vi "Extract Project Strings.vi"(8 "error in (no error)":errorcluster, 11 "New Project Wizard in":refnum<class "Update Project Wizard.lvclass">) -> (0 "error out":errorcluster, 3 "New Project Wizard out":refnum<class "Update Project Wizard.lvclass">)   [LabVIEW 2013, in "SET Project Editor.lvlib" / "Update Project Wizard.lvclass"]
uses:
  Update Project Wizard.lvclass
  Update Project Wizard.lvclass/Update Project Wizard.ctl
  SET Project Data/Project Data Class/Project Data.lvclass
  SET Project Data/Resource Data Class/Resource Data.lvclass
  Lib/Printf/Messages/General/LV_Printf Msg.lvclass
  SET Project Data/VI Class/VI Data.lvclass
  SET Project Data/Menu Class/Menu Data.lvclass
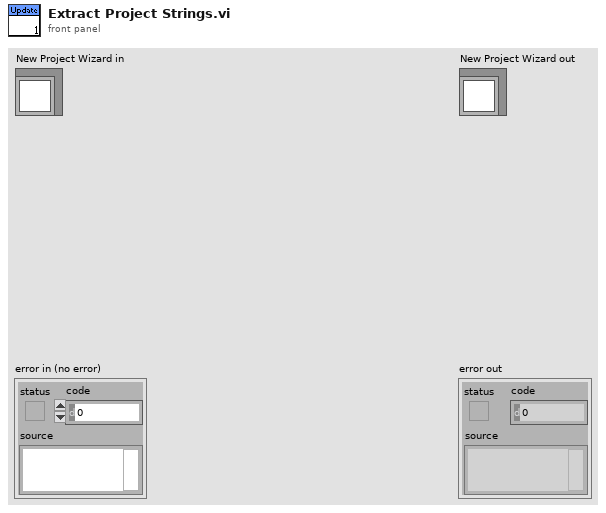
[diagram p1: front panel]
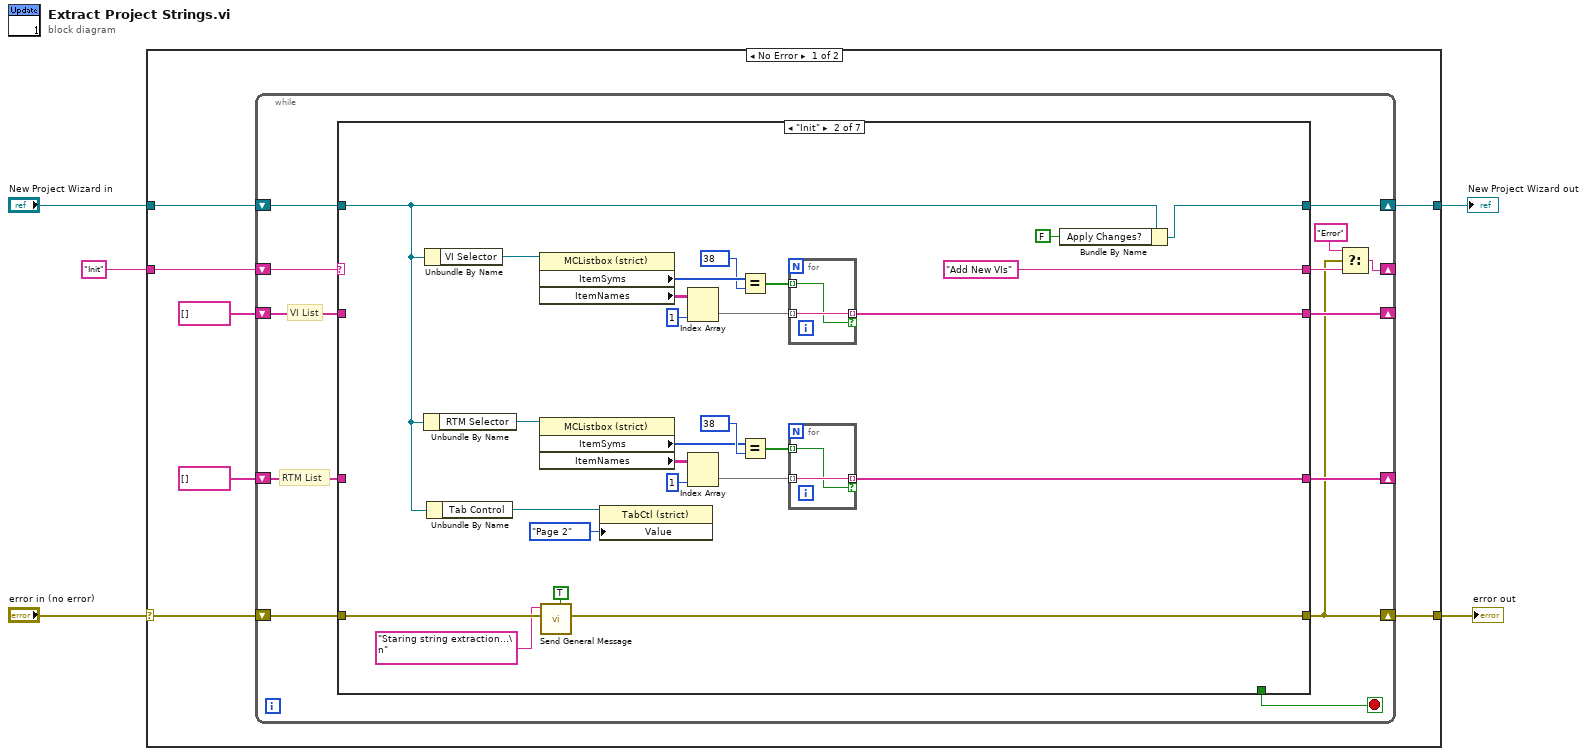
[diagram p0: block diagram]
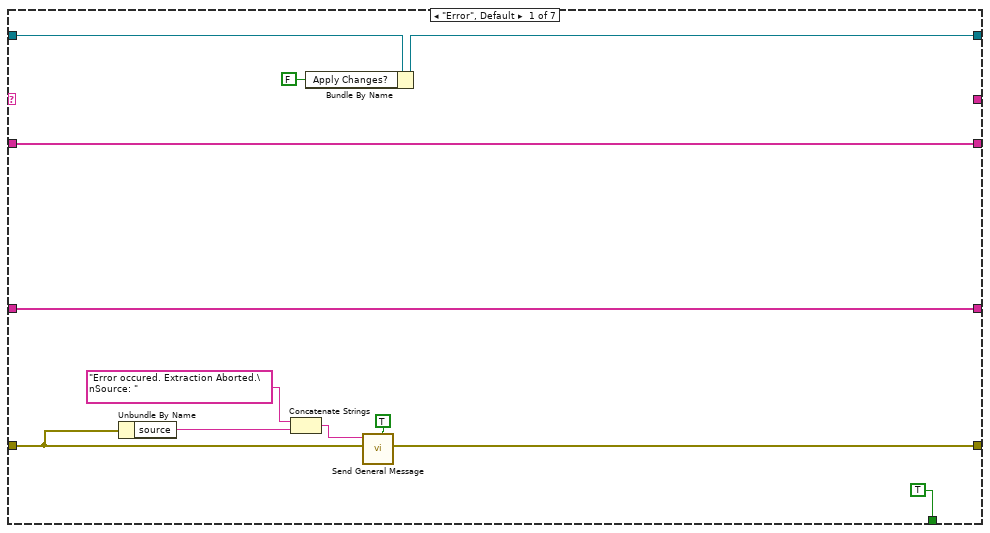
[diagram p2: hidden frame]
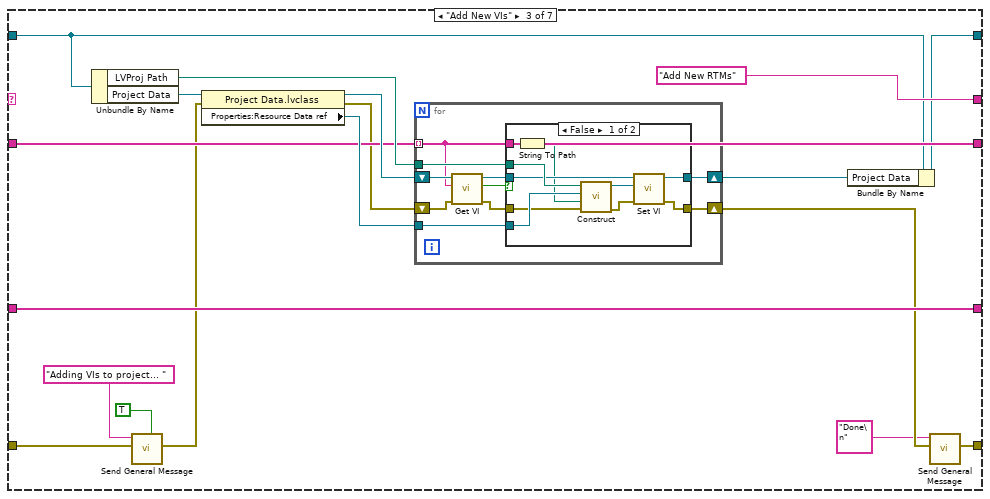
[diagram p3: hidden frame]
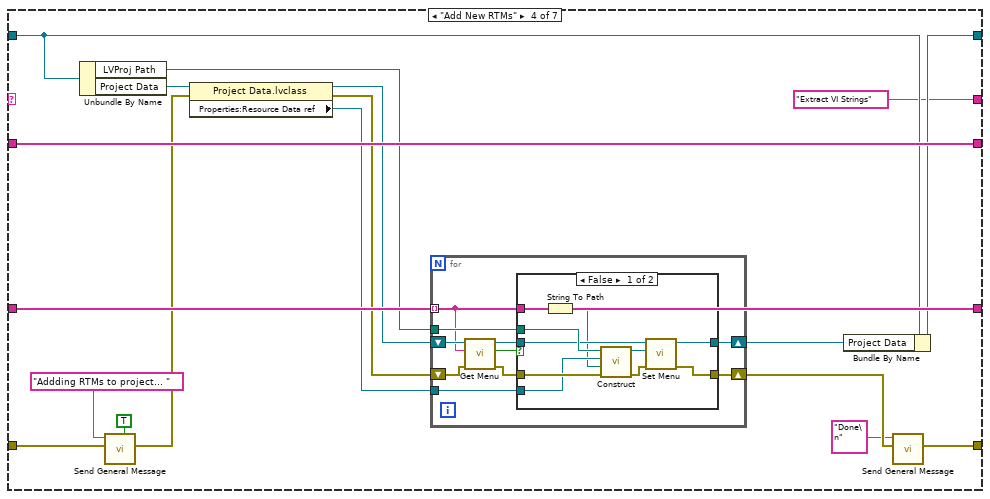
[diagram p5: hidden frame]
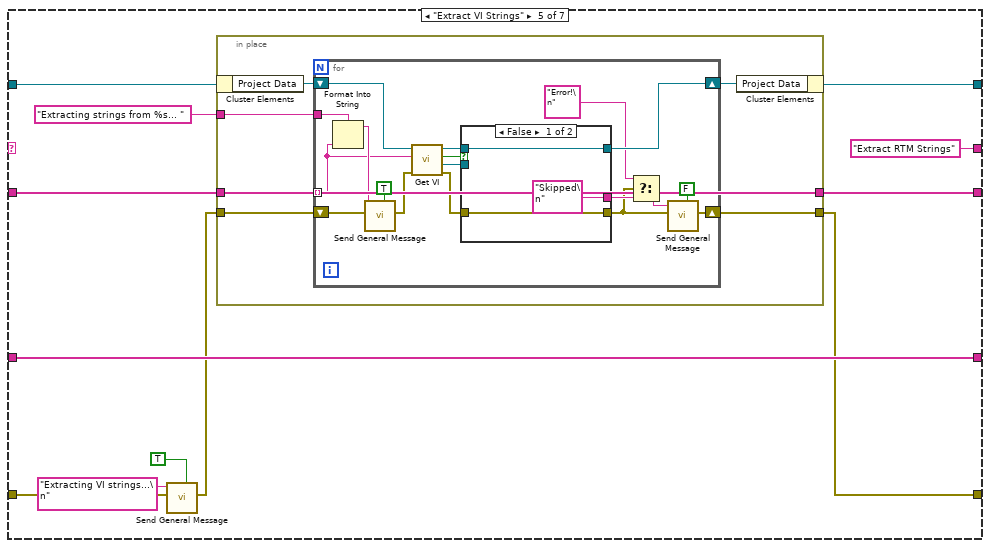
[diagram p7: hidden frame]
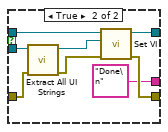
[diagram p8: hidden frame]
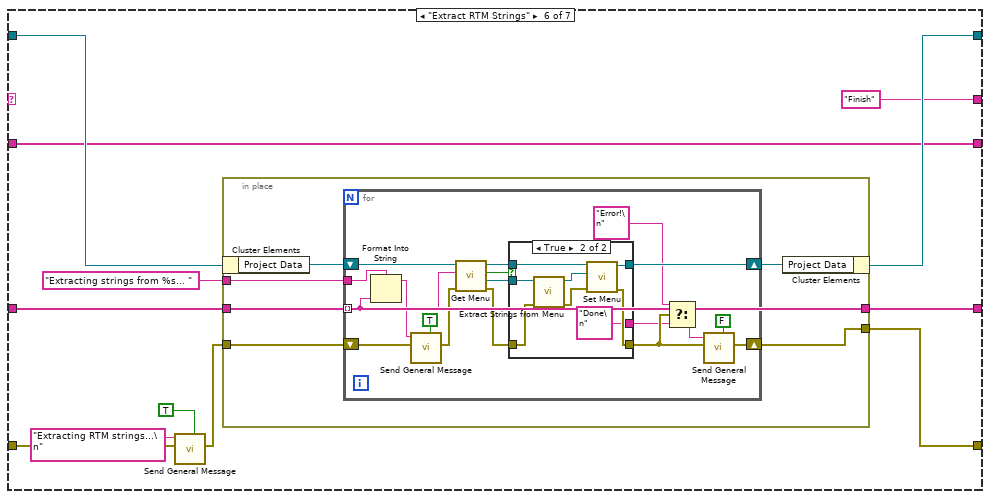
[diagram p9: hidden frame]
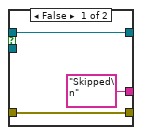
[diagram p10: hidden frame]
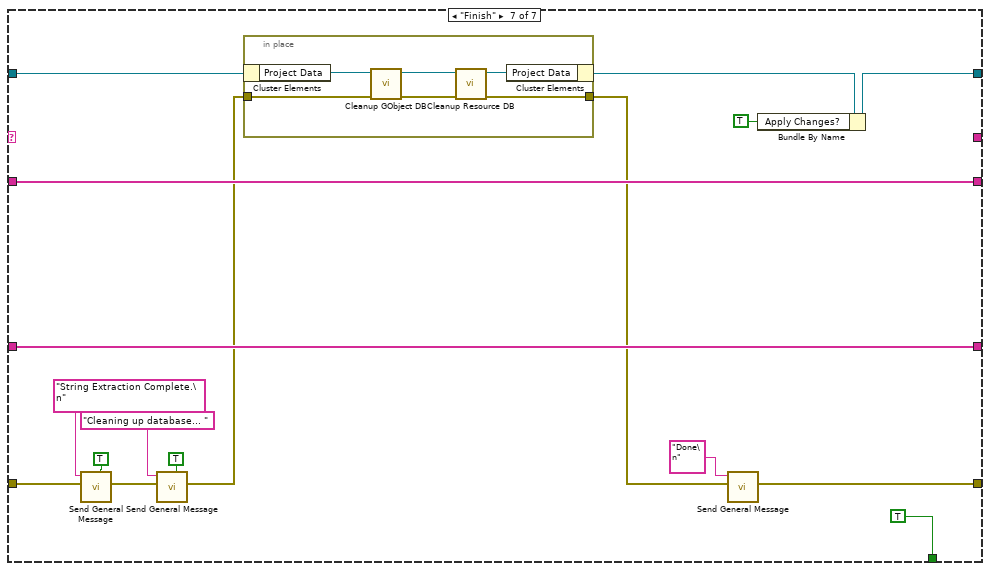
[diagram p11: hidden frame]
diagram:
  n1 = case shown="No Error" "error in (no error)" {
    selector: "error in (no error)" -> [w7 w266]
    tunnel: [w6 w266] -> w1
    tunnel: [w8 w265] -> w2
    tunnel: "New Project Wizard in" -> [w12 w265]
    tunnel: "Init" -> [w11 _]
    frame No Error {
      n2 = while {
        shift-right: [w14] -> _
        shift-left: w11 -> [w25]
        shift-right: [w19] -> w8
        shift-left: w12 -> [w24]
        shift-right: [w23] -> _
        shift-left: string[] [] -> [w22]
        shift-right: [w21] -> _
        shift-left: string[] [] -> [w20]
        shift-right: [w15] -> w6
        shift-left: w7 -> [w17]
        stop <- w18 stop-if-true
        # "RTM List"
        # "VI List"
        n3 = case shown="\"Init\"" w25 {
          tunnel: w24 -> [w28 w38 w78 w118 w159 w206 w255]
          tunnel: [w37 w56 w80 w123 w157 w201 w258] -> w23
          tunnel: w22 -> [w37 _ w80 w123 w158 w201 w258]
          tunnel: [w36 w48 w81 w124 w154 w202 w257] -> w21
          tunnel: w20 -> [w36 _ w81 w124 w154 w203 w257]
          tunnel: [w27 w39 w77 w117 w156 w205 w243] -> w19
          tunnel: [_ "Add New VIs" "Add New RTMs" "Extract VI Strings" "Extract RTM Strings" "Finish" _] -> w16
          tunnel: [TRUE _ _ _ _ _ TRUE] -> w18
          tunnel: w17 -> [w32 w44 w74 w114 w152 w197 w254]
          tunnel: [w33 w41 w70 w110 w153 w200 w246] -> w15
          frame "Error", Default {
            n4 = Unbundle By Name(w32) -> ("source"=w30:string)
            n5 = Concatenate Strings("Error occured. Extraction Aborted.\nSource: ", w30) -> (w29:string)
            n6 = Bundle By Name(cluster=w28, "Apply Changes?"=FALSE) -> (w27:refnum<class "Update Project Wizard.lvclass">)
            n7 = call "Send General Message.vi"("Timestamp in message? (F)"=TRUE, "error in (no error)"=w32, "Message"=w29) -> ("error out"=w33:errorcluster)  [unwired: 8 in]
          }
          frame "Init" {
            n8 = Unbundle By Name(w38) -> ("RTM Selector"=w49:refnum<vi>)
            n9 = Unbundle By Name(w38) -> ("VI Selector"=w59:refnum<vi>)
            n10 = Unbundle By Name(w38) -> ("Tab Control"=w46:refnum<vi>)
            n11 = property class="MCListbox (strict)"(reference=w59) -> ("ItemSyms"=w61:i32[], "ItemNames"=w62:string[][])  [unwired: 1 in, 2 out]
            n12 = property class="MCListbox (strict)"(reference=w49) -> ("ItemSyms"=w52:i32[], "ItemNames"=w51:string[][])  [unwired: 1 in, 2 out]
            n13 = call "Send General Message.vi"("Timestamp in message? (F)"=TRUE, "error in (no error)"=w44, "Message"="Staring string extraction...\n" ("Status")) -> ("error out"=w41:errorcluster)  [unwired: 8 in]
            n14 = property class="TabCtl (strict)"(reference=w46, "Value"=enum32{"Page 1", "Page 2"}."Page 2") -> ()  [unwired: 1 in, 2 out]
            n15 = Index Array(array=w62, index (col)=1 ("disabled index (col)")) -> (element=w58:string[])  [unwired: 1 in]
            n16 = Index Array(array=w51, index (col)=1 ("disabled index (col)")) -> (element=w54:string[])  [unwired: 1 in]
            n17 = Equal?(x=w61, y=38) -> (x = y?=w57:bool[])
            n18 = Equal?(x=w52, y=38) -> (x = y?=w55:bool[])
            n19 = for {
              tunnel: w58 -> [w67] mode=indexing
              tunnel: w57 -> [w66] mode=indexing
              tunnel: [w67] -> w56 mode=indexing if=w66
            }
            n20 = for {
              tunnel: w54 -> [w65] mode=indexing
              tunnel: w55 -> [w64] mode=indexing
              tunnel: [w65] -> w48 mode=indexing if=w64
            }
            n21 = Bundle By Name(cluster=w38, "Apply Changes?"=FALSE) -> (w39:refnum<class "Update Project Wizard.lvclass">)
          }
          frame "Add New VIs" {
            n22 = Unbundle By Name(w78) -> ("LVProj Path"=w84:path, "Project Data"=w85:refnum<class "Project Data.lvclass">)
            n23 = call "Send General Message.vi"("Timestamp in message? (F)"=TRUE ("Timestamp in message? (T)"), "error in (no error)"=w74, "Message"="Adding VIs to project... ") -> ("error out"=w73:errorcluster)  [unwired: 8 in]
            n24 = property class="Project Data.lvclass"(reference=w85, error in=w73) -> (reference out=w83:refnum<class "Project Data.lvclass">, error out=w75:errorcluster, "Properties:Resource Data ref"=w82:refnum<data-value>)
            n25 = for {
              shift-right: [w94] -> w76
              shift-left: w83 -> [w95]
              shift-right: [w93] -> w71
              shift-left: w75 -> [w91]
              tunnel: w82 -> [w92]
              tunnel: w84 -> [w90]
              tunnel: w80 -> [w89] mode=indexing
              n26 = call-dynamic "Get VI.vi"("error in (no error)"=w91, "VI Path (Relative)"=w89, "ProjectData in"=w95) -> ("error out"=w87:errorcluster, "found"=w86:bool, "ProjectData out"=w88:refnum<class "Project Data.lvclass">)  [unwired: 5 in, 1 out]
              n27 = case shown="False" w86 {
                tunnel: [w105 w107] -> w94
                tunnel: [w104 w106] -> w93
                tunnel: w92 -> [w101 _]
                tunnel: w90 -> [w100 _]
                tunnel: w88 -> [w99 w107]
                tunnel: w89 -> [w98 _]
                tunnel: w87 -> [w96 w106]
                frame False {
                  n28 = String To Path(string=w98) -> (path=w97:path)
                  n29 = call "Construct.vi"("error in (no error)"=w96, "VI Path (Relative)"=w97, "Resource Data ref"=w101, "LVProject File Path (Absolute)"=w100) -> ("error out"=w103:errorcluster, "VI Data out"=w102:refnum<class "VI Data.lvclass">)  [unwired: 6 in]
                  n30 = call-dynamic "Set VI.vi"("error in (no error)"=w103, "VI Data in"=w102, "ProjectData in"=w99) -> ("error out"=w104:errorcluster, "ProjectData out"=w105:refnum<class "Project Data.lvclass">)  [unwired: 6 in, 1 out]
                }
                frame True {
                }
              }
            }
            n31 = Bundle By Name(cluster=w78, "Project Data"=w76) -> (w77:refnum<class "Update Project Wizard.lvclass">)
            n32 = call "Send General Message.vi"("error in (no error)"=w71, "Message"="Done\n") -> ("error out"=w70:errorcluster)  [unwired: 9 in]
          }
          frame "Add New RTMs" {
            n33 = Unbundle By Name(w118) -> ("LVProj Path"=w122:path, "Project Data"=w125:refnum<class "Project Data.lvclass">)
            n34 = call "Send General Message.vi"("Timestamp in message? (F)"=TRUE, "error in (no error)"=w114, "Message"="Addding RTMs to project... ") -> ("error out"=w113:errorcluster)  [unwired: 8 in]
            n35 = property class="Project Data.lvclass"(reference=w125, error in=w113) -> (reference out=w121:refnum<class "Project Data.lvclass">, error out=w119:errorcluster, "Properties:Resource Data ref"=w120:refnum<data-value>)
            n36 = for {
              shift-right: [w134] -> w116
              shift-left: w121 -> [w135]
              shift-right: [w133] -> w109
              shift-left: w119 -> [w131]
              tunnel: w120 -> [w132]
              tunnel: w122 -> [w130]
              tunnel: w124 -> [w129] mode=indexing
              n37 = call-dynamic "Get Menu.vi"("error in (no error)"=w131, "Menu Path (Relative)"=w129, "ProjectData in"=w135) -> ("error out"=w126:errorcluster, "found"=w127:bool, "ProjectData out"=w128:refnum<class "Project Data.lvclass">)  [unwired: 5 in, 1 out]
              n38 = case shown="False" w127 {
                tunnel: w126 -> [w145 w146]
                tunnel: w132 -> [w144 _]
                tunnel: w130 -> [w143 _]
                tunnel: w128 -> [w142 w147]
                tunnel: [w141 w147] -> w134
                tunnel: [w139 w146] -> w133
                tunnel: w129 -> [w137 _]
                frame False {
                  n39 = String To Path(string=w137) -> (path=w136:path)
                  n40 = call "Construct.vi"("error in (no error)"=w145, "Menu Path (Relative)"=w136, "Resource Data ref"=w144, "LVProject File Path"=w143) -> ("error out"=w138:errorcluster, "Menu Data out"=w140:refnum<class "Menu Data.lvclass">)  [unwired: 6 in]
                  n41 = call-dynamic "Set Menu.vi"("error in (no error)"=w138, "RTM Data in"=w140, "ProjectData in"=w142) -> ("error out"=w139:errorcluster, "ProjectData out"=w141:refnum<class "Project Data.lvclass">)  [unwired: 6 in, 1 out]
                }
                frame True {
                }
              }
            }
            n42 = Bundle By Name(cluster=w118, "Project Data"=w116) -> (w117:refnum<class "Update Project Wizard.lvclass">)
            n43 = call "Send General Message.vi"("error in (no error)"=w109, "Message"="Done\n") -> ("error out"=w110:errorcluster)  [unwired: 9 in]
          }
          frame "Extract VI Strings" {
            n44 = call "Send General Message.vi"("Timestamp in message? (F)"=TRUE, "error in (no error)"=w152, "Message"="Extracting VI strings...\n") -> ("error out"=w151:errorcluster)  [unwired: 8 in]
            n45 = in-place {
              in-place-border: w158 -> [w163]
              in-place-border: [w163] -> w157
              in-place-border: w151 -> [w162]
              in-place-border: [w161] -> w153
              in-place-border: "Extracting strings from %s... " -> [w160]
              n46 = in-place-cluster #1(w159) -> ("Project Data"=w165:refnum<class "Project Data.lvclass">)
              n47 = for {
                tunnel: w163 -> [w166] mode=indexing
                shift-right: [w177] -> w161
                shift-left: w162 -> [w171]
                shift-right: [w178] -> w164
                shift-left: w165 -> [w183]
                tunnel: w160 -> [w168]
                n48 = Format Into String(format string=w168, w166) -> (resulting string=w167:string)  [unwired: 2 in, 1 out]
                n49 = call "Send General Message.vi"("Timestamp in message? (F)"=TRUE, "error in (no error)"=w171, "Message"=w167) -> ("error out"=w170:errorcluster)  [unwired: 8 in]
                n50 = call-dynamic "Get VI.vi"("error in (no error)"=w170, "VI Path (Relative)"=w166, "ProjectData in"=w183) -> ("error out"=w181:errorcluster, "VI Data out"=w182:refnum<class "VI Data.lvclass">, "found"=w179:bool, "ProjectData out"=w180:refnum<class "Project Data.lvclass">)  [unwired: 5 in]
                n51 = case shown="False" w179 {
                  tunnel: w182 -> [_ w194]
                  tunnel: w181 -> [w186 w193]
                  tunnel: w180 -> [w185 w192]
                  tunnel: [w186 w189] -> w172
                  tunnel: [w185 w188] -> w178
                  tunnel: ["Skipped\n" "Done\n"] -> w174
                  frame False {
                  }
                  frame True {
                    n52 = call "Extract All UI Strings.vi"("error in (no error)"=w193, "LanguageData in"=w194) -> ("error out"=w190:errorcluster, "LanguageData out"=w191:refnum<class "VI Data.lvclass">)  [unwired: 8 in]
                    n53 = call-dynamic "Set VI.vi"("error in (no error)"=w190, "VI Data in"=w191, "ProjectData in"=w192) -> ("error out"=w189:errorcluster, "ProjectData out"=w188:refnum<class "Project Data.lvclass">)  [unwired: 6 in, 1 out]
                  }
                }
                n54 = Select(t="Error!\n", s=w172, f=w174) -> (s? t:f=w173:string)
                n55 = call "Send General Message.vi"("Timestamp in message? (F)"=FALSE, "error in (no error)"=w172, "Message"=w173) -> ("error out"=w177:errorcluster)  [unwired: 8 in]
              }
              n56 = in-place-cluster #1("Project Data"=w164) -> (w156:refnum<class "Update Project Wizard.lvclass">)
            }
          }
          frame "Extract RTM Strings" {
            n57 = call "Send General Message.vi"("Timestamp in message? (F)"=TRUE, "error in (no error)"=w197, "Message"="Extracting RTM strings...\n") -> ("error out"=w196:errorcluster)  [unwired: 8 in]
            n58 = in-place {
              in-place-border: w203 -> [w210]
              in-place-border: [w210] -> w202
              in-place-border: w196 -> [w209]
              in-place-border: [w208] -> w200
              in-place-border: "Extracting strings from %s... " -> [w207]
              n59 = in-place-cluster #2(w206) -> ("Project Data"=w212:refnum<class "Project Data.lvclass">)
              n60 = for {
                tunnel: w210 -> [w224] mode=indexing
                shift-right: [w216] -> w208
                shift-left: w209 -> [w222]
                shift-right: [w230] -> w211
                shift-left: w212 -> [w229]
                tunnel: w207 -> [w213]
                n61 = Format Into String(format string=w213, w224) -> (resulting string=w220:string)  [unwired: 2 in, 1 out]
                n62 = call "Send General Message.vi"("Timestamp in message? (F)"=TRUE, "error in (no error)"=w222, "Message"=w220) -> ("error out"=w221:errorcluster)  [unwired: 8 in]
                n63 = call-dynamic "Get Menu.vi"("error in (no error)"=w221, "Menu Path (Relative)"=w224, "ProjectData in"=w229) -> ("error out"=w228:errorcluster, "Menu Data out"=w227:refnum<class "Menu Data.lvclass">, "found"=w226:bool, "ProjectData out"=w225:refnum<class "Project Data.lvclass">)  [unwired: 5 in]
                n64 = case shown="True" w226 {
                  tunnel: w227 -> [_ w241]
                  tunnel: w228 -> [w233 w235]
                  tunnel: w225 -> [w232 w240]
                  tunnel: [w233 w238] -> w217
                  tunnel: [w232 w239] -> w230
                  tunnel: ["Skipped\n" "Done\n"] -> w214
                  frame False {
                  }
                  frame True {
                    n65 = call "Extract Strings from Menu.vi"("error in (no error)"=w235, "Object in"=w241) -> ("error out"=w237:errorcluster, "Object out"=w236:refnum<class "Menu Data.lvclass">)  [unwired: 8 in]
                    n66 = call-dynamic "Set Menu.vi"("error in (no error)"=w237, "RTM Data in"=w236, "ProjectData in"=w240) -> ("error out"=w238:errorcluster, "ProjectData out"=w239:refnum<class "Project Data.lvclass">)  [unwired: 6 in, 1 out]
                  }
                }
                n67 = Select(t="Error!\n", s=w217, f=w214) -> (s? t:f=w218:string)
                n68 = call "Send General Message.vi"("Timestamp in message? (F)"=FALSE, "error in (no error)"=w217, "Message"=w218) -> ("error out"=w216:errorcluster)  [unwired: 8 in]
              }
              n69 = in-place-cluster #2("Project Data"=w211) -> (w205:refnum<class "Update Project Wizard.lvclass">)
            }
          }
          frame "Finish" {
            n70 = call "Send General Message.vi"("Timestamp in message? (F)"=TRUE, "error in (no error)"=w254, "Message"="String Extraction Complete.\n") -> ("error out"=w249:errorcluster)  [unwired: 8 in]
            n71 = call "Send General Message.vi"("Timestamp in message? (F)"=TRUE, "error in (no error)"=w249, "Message"="Cleaning up database... ") -> ("error out"=w248:errorcluster)  [unwired: 8 in]
            n72 = in-place {
              in-place-border: w248 -> [w260]
              in-place-border: [w259] -> w247
              n73 = in-place-cluster #3(w255) -> ("Project Data"=w262:refnum<class "Project Data.lvclass">)
              n74 = call "Cleanup GObject DB.vi"("error in (no error)"=w260, "Project Data in"=w262) -> ("error out"=w263:errorcluster, "Project Data out"=w264:refnum<class "Project Data.lvclass">)  [unwired: 8 in]
              n75 = call-dynamic "Cleanup Resource DB.vi"("error in (no error)"=w263, "ProjectData in"=w264) -> ("error out"=w259:errorcluster, "ProjectData out"=w261:refnum<class "Project Data.lvclass">)  [unwired: 8 in]
              n76 = in-place-cluster #3("Project Data"=w261) -> (w244:refnum<class "Update Project Wizard.lvclass">)
            }
            n77 = call "Send General Message.vi"("error in (no error)"=w247, "Message"="Done\n") -> ("error out"=w246:errorcluster)  [unwired: 9 in]
            n78 = Bundle By Name(cluster=w244, "Apply Changes?"=TRUE) -> (w243:refnum<class "Update Project Wizard.lvclass">)
          }
        }
        n79 = Select(t="Error", s=w15, f=w16) -> (s? t:f=w14:string)
      }
    }
    frame Error {
    }
  }
  "error out" <- w1
  "New Project Wizard out" <- w2
